vi "flattenTimeToXML_Scalar.vi"(8 "error in (no error)":errorcluster, 9 "timeUnitInXML":T1, 10 "timeAgain":variant, 11 "time":dbl[unit]) -> (0 "error out":errorcluster, 3 "xmlString":string)   [LabVIEW 2016, in "UnitsAndXML.lvlib"]
uses:
  <userlib>/Common/UnitsAndXML/UnitsAndXML.lvlib
  <userlib>/Common/UnitsAndXML/FlattenItemWithUnitToXML/FlattenTimeToXML/TimeUnit.ctl
  <vilib>/Utility/VariantDataType/VariantType.lvlib
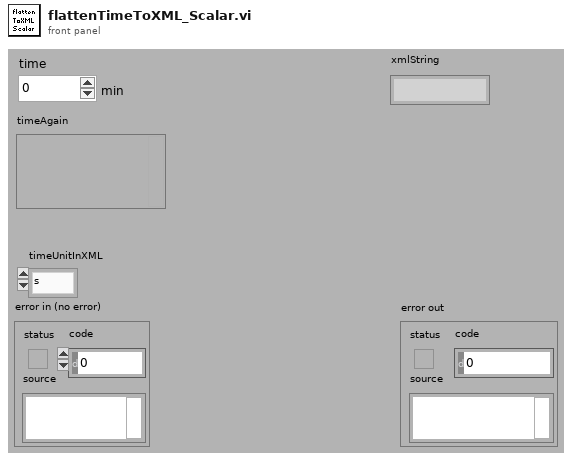
[diagram p1: front panel]
types:
  T1 = typedef "UnitsAndXML.lvlib/TimeUnit.ctl" = enum16{"s", "d", "h", "min", "a"}
  T2 = typedef "VariantType.lvlib/Type.ctl" = enum8{"Invalid Type", "Void", "I8", "I16", "I32", "I64", "U8", "U16", "U32", "U64", "Single Float", "Double Float", "Extended Float", "Single Complex", "Double Complex", "Extended Complex", "Enum U8", "Enum U16", "Enum U32", "Enum U64", "Single Float With Unit", "Double Float With Unit", "Extended Float With Unit", "Single Complex with Unit", "Double Complex with Unit", "Extended Complex with Unit", "Boolean", "String", "Path", "Picture", "Tag", "Array", "Cluster", "Variant", "LV Variant", "Waveform", "Timestamp", "Digital Waveform", "Digital Data", "ExpressData", "Refnum", "External Data", "VI", "Poly VI", "LabVIEW Class Instance", "Fixed Point"}
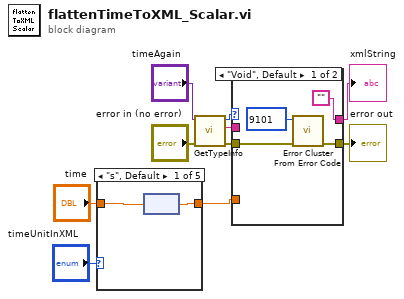
[diagram p0: block diagram]
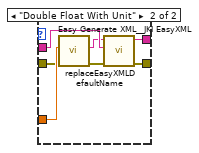
[diagram p2: hidden frame]
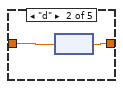
[diagram p3: hidden frame]
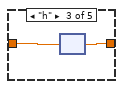
[diagram p4: hidden frame]
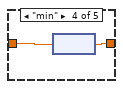
[diagram p5: hidden frame]
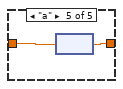
[diagram p6: hidden frame]
diagram:
  n1 = case shown="\"s\", Default" "timeUnitInXML" {
    tunnel: "time" -> [w12 w14 w16 w18 w20]
    tunnel: [w11 w13 w15 w17 w19] -> w10
    frame "s", Default {
      n2 = node(w12) -> (w11:dbl)
    }
    frame "d" {
      n3 = node(w14) -> (w13:dbl)
    }
    frame "h" {
      n4 = node(w16) -> (w15:dbl)
    }
    frame "min" {
      n5 = node(w18) -> (w17:dbl)
    }
    frame "a" {
      n6 = node(w20) -> (w19:dbl)
    }
  }
  n7 = call <vilib>:"GetTypeInfo.vi"("error in (no error)"="error in (no error)", "Variant"="timeAgain") -> ("error out"=w2:errorcluster, "Name"=w1:string, "Type Enum"=w3:T2)  [unwired: 5 in, 2 out]
  n8 = case shown="\"Void\", Default" w3 {
    tunnel: w10 -> [_ w31]
    tunnel: ["" w30] -> w7
    tunnel: [w23 w29] -> w6
    tunnel: w2 -> [w21 w26]
    tunnel: w1 -> [_ w28]
    frame "Void", Default {
      n9 = call <vilib>:"Error Cluster From Error Code.vi"("error in (no error)"=w21, "error code (0)"=9101) -> ("error out"=w23:errorcluster)  [unwired: 7 in]
    }
    frame "Double Float With Unit" {
      n10 = call <vilib>:"Easy Generate XML__JKI EasyXML.vi"("error in (no error)"=w26, "LabVIEW Data"=w31) -> ("error out"=w25:errorcluster, "XML String"=w27:string)  [unwired: 8 in]
      n11 = call <userlib>:"replaceEasyXMLDefaultName.vi"("error in"=w25, "desiredName"=w28, "easyXMLStringWithDefaultNames"=w27) -> ("error out"=w29:errorcluster, "xmlString"=w30:string)  [unwired: 7 in]
    }
  }
  "xmlString" <- w7
  "error out" <- w6
